vi "DT_Hold_Open.vi"   [LabVIEW 2011]
uses:
  <userlib>/LV-Link3/DtLvLink_32.dll
panel:
  # "This Vi holds an instance of  LV-Link open"
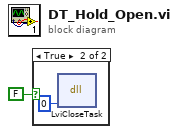
[diagram p0: block diagram]
diagram:
  n1 = case shown="True" FALSE {
    frame False {
    }
    frame True {
      n2 = dll-call lib="C:/Program Files/National Instruments/LabVIEW 2011/user.lib/LV-Link3/DtLvLink_32.*" fn="LviCloseTask"("TaskRef"=0) -> ()  [unwired: 5 in, 2 out]
    }
  }
